vi "InserNewLibraryRange.vi"(6 "Size":i32, 8 "ErrorIn":errorcluster caption="Error In(no Error)", 9 "StartRange":i32, 10 "Library":string, 11 "ReferenceIn":refnum<class "ErrorDefinitionSQLite.lvclass"> caption="Reference In") -> (0 "ErrorOut":errorcluster caption="Error Out", 3 "ReferenceOut":refnum<class "ErrorDefinitionSQLite.lvclass"> caption="Reference Out")   [LabVIEW 2018, in "ErrorDefinitionSQLite.lvclass"]
uses:
  ErrorDefinitionSQLite.lvclass
  <vilib>/drjdpowell/SQLite Library/SQL Connection/Execute SQL.vi
  <vilib>/drjdpowell/SQLite Library/SQLite.lvlib
  <vilib>/drjdpowell/SQLite Library/SQL Connection/Connection.lvclass
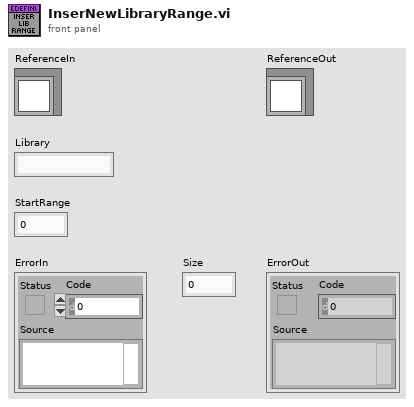
[diagram p1: front panel]
types:
  T1 = typedef "ErrorDefinitionSQLite.lvclass/ObjectAttributes.ctl" = cluster{"Path":path, "SQLiteRef":refnum<class "Connection.lvclass">, "EndOfRange":i32, "DefaultLibrarySize":i32, "StartOfRange":i32}
  T2 = cluster{"Library":string, string, string, "App.UserName":string}
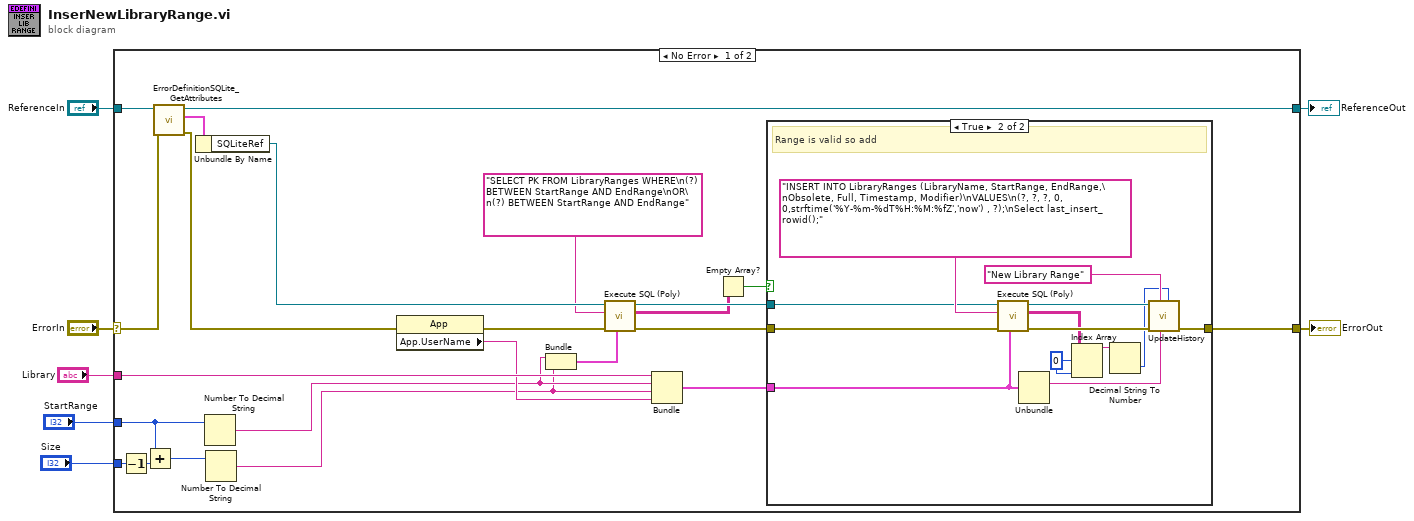
[diagram p0: block diagram]
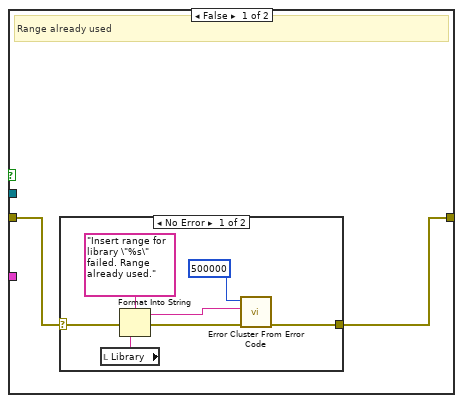
[diagram p2: hidden frame]
diagram:
  n1 = case shown="No Error" "ErrorIn" {
    selector: "ErrorIn" -> [w30 w55]
    tunnel: [w24 w55] -> w6
    tunnel: [w28 w54] -> w4
    tunnel: "ReferenceIn" -> [w29 w54]
    tunnel: "Library" -> [w23 _]
    tunnel: "Size" -> [w22 _]
    tunnel: "StartRange" -> [w21 _]
    frame No Error {
      n2 = Decrement(x=w22) -> (x-1=w8:i32)
      n3 = Add(x=w21, y=w8) -> (x+y=w20:i32)
      n4 = call "ErrorDefinitionSQLite_GetAttributes.vi"("ErrorIn"=w30, "Reference in"=w29) -> ("ErrorOut"=w25:errorcluster, "Data"=w27:T1, "Reference out"=w28:refnum<class "ErrorDefinitionSQLite.lvclass">)  [unwired: 6 in, 1 out]
      n5 = Unbundle By Name(w27) -> ("SQLiteRef"=w26:refnum<class "Connection.lvclass">)
      n6 = Number To Decimal String(number=w21) -> (decimal integer string=w13:string)  [unwired: 1 in]
      n7 = Number To Decimal String(number=w20) -> (decimal integer string=w12:string)  [unwired: 1 in]
      n8 = property class="App"(error in=w25) -> (error out=w17:errorcluster, "App.UserName"=w19:string)  [unwired: 1 in, 1 out]
      n9 = Bundle(w13, w12) -> (w11:cluster{string, string})  [unwired: 1 in]
      n10 = call-poly <vilib>:"Execute SQL (Poly).vi"("Parameter(s)"=w11, "error in (no error)"=w17, "SQL"="SELECT PK FROM LibraryRanges WHERE\n(?) BETWEEN StartRange AND EndRange\nOR\n(?) BETWEEN StartRange AND EndRange", "SQLite Connection in"=w26) -> ("error out"=w15:errorcluster, "Result Set"=w10:string[][], "SQLite Connection"=w16:refnum<class "Connection.lvclass">)  [unwired: 4 in, 1 out]
      n11 = Bundle("Library"=w23, w13, w12, "App.UserName"=w19) -> (w18:T2)  [unwired: 1 in]
      n12 = Empty Array?(array=w10) -> (empty?=w9:bool)
      n13 = case shown="True" w9 {
        tunnel: [w31 w49] -> w24
        tunnel: w18 -> [_ w46]
        tunnel: w16 -> [_ w51]
        tunnel: w15 -> [w32 w50]
        frame False {
          # "Range already used"
          n14 = case shown="No Error" w32 {
            selector: w32 -> [w39 w40]
            tunnel: [w38 w40] -> w31
            frame No Error {
              n15 = local read "Library"() -> (w34:string)
              n16 = Format Into String(format string="Insert range for library \"%s\" failed. Range already used." ("error message (\"\")"), error in=w39, w34) -> (resulting string=w33:string, error out=w36:errorcluster)  [unwired: 1 in]
              n17 = call <vilib>:"Error Cluster From Error Code.vi"("error in (no error)"=w36, "error message (\"\")"=w33, "error code (0)"=500000) -> ("error out"=w38:errorcluster)  [unwired: 6 in]
            }
            frame Error {
            }
          }
        }
        frame True {
          w43 = 0 ("index (row)")
          # "Range is valid so add"
          n18 = call-poly <vilib>:"Execute SQL (Poly).vi"("Parameter(s)"=w46, "error in (no error)"=w50, "SQL"="INSERT INTO LibraryRanges (LibraryName, StartRange, EndRange,\nObsolete, Full, Timestamp, Modifier)\nVALUES\n(?, ?, ?, 0, 0,strftime('%Y-%m-%dT%H:%M:%fZ','now') , ?);\nSelect last_insert_rowid();", "SQLite Connection in"=w51) -> ("error out"=w53:errorcluster, "Result Set"=w44:string[][], "SQLite Connection"=w48:refnum<class "Connection.lvclass">)  [unwired: 4 in, 1 out]
          n19 = Unbundle(w46) -> ("Library"=w45:string)  [unwired: 3 out]
          n20 = Index Array(array=w44, index (row)=w43, index (col)=w43) -> (element=w42:string)
          n21 = Decimal String To Number(string=w42) -> (number=w41:i32)  [unwired: 2 in, 1 out]
          n22 = call "UpdateHistory.vi"("LibraryPK"=w41, "Library"=w45, "Action"="New Library Range", "error in (no error)"=w53, "Connection in"=w48) -> ("error out"=w49:errorcluster)  [unwired: 5 in, 1 out]
        }
      }
    }
    frame Error {
    }
  }
  "ErrorOut" <- w6
  "ReferenceOut" <- w4
